vi "Property Name_Dots and Indents.vi"(11 "Property":string) -> (3 "Cluster":T1)   [LabVIEW 2023]
doc: "Bare property is when you have a subproperty (Bounds:Height) and you want just \"Height\"."
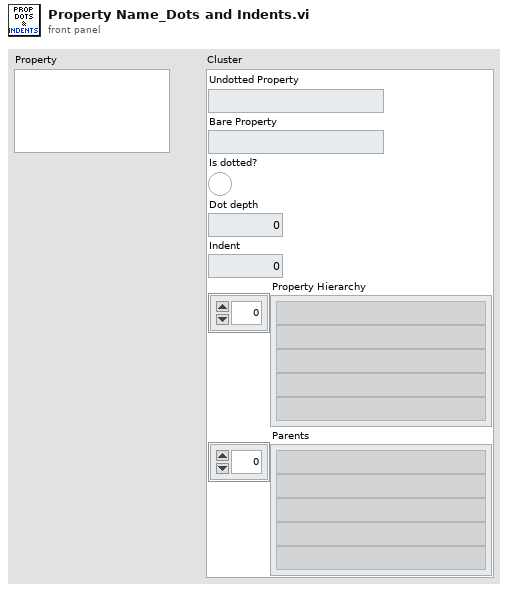
[diagram p1: front panel]
types:
  T1 = cluster{"Undotted Property":string, "Bare Property":string, "Is dotted?":bool, "Dot depth":i32, "Indent":i32, "Property Hierarchy":string[], "Parents":string[]}
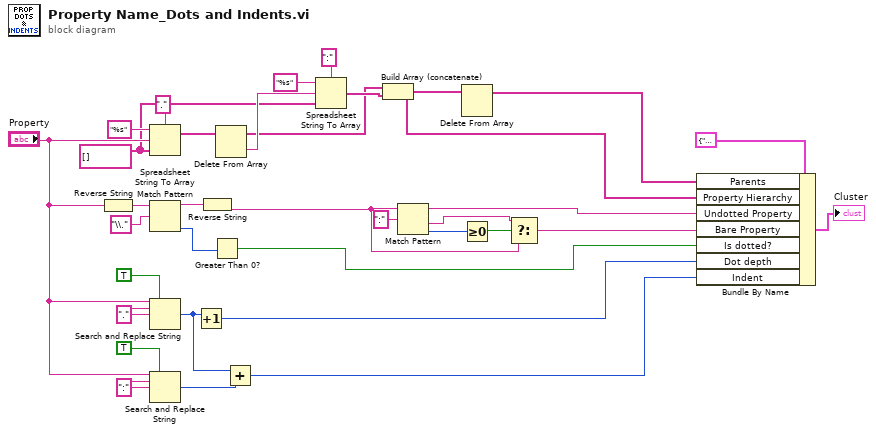
[diagram p0: block diagram]
diagram:
  w24 = ":" ("regular expression")
  w4 = string[] [] ("format string")
  w29 = "." ("regular expression")
  n1 = Reverse String(1:"Property") -> (0:w33:string)
  n2 = Spreadsheet String To Array(delimiter (Tab)=".", format string="%s", spreadsheet string="Property", array type (2D Dbl)=w4) -> (array=w8:string[])
  n3 = Match Pattern(string=w33, regular expression="\\.") -> (before substring=w31:string, offset past match=w30:i32)  [unwired: 1 in, 2 out]
  n4 = Search and Replace String(replace all?=TRUE ("replace all? (F)"), input string="Property", search string=w29, replace string=w29) -> (number of replacements=w23:i32)  [unwired: 4 in, 3 out]
  n5 = Search and Replace String(replace all?=TRUE ("replace all? (F)"), input string="Property", search string=w24, replace string=w24) -> (number of replacements=w22:i32)  [unwired: 4 in, 3 out]
  n6 = Increment(x=w23) -> (x+1=w11:i32)
  n7 = Reverse String(1:w31) -> (0:w13:string)
  n8 = Greater Than 0?(x=w30) -> (x > 0?=w12:bool)
  n9 = Delete From Array(array=w8) -> (deleted portion=w7:string, array with subset deleted=w3:string[])  [unwired: 2 in]
  n10 = Add(x=w23, y=w22) -> (x+y=w10:i32)
  n11 = Spreadsheet String To Array(delimiter (Tab)=":", format string="%s", spreadsheet string=w7, array type (2D Dbl)=w4) -> (array=w5:string[])
  n12 = Build Array (concatenate)(w3, w5) -> (w2:string[])
  n13 = Match Pattern(string=w13, regular expression=":") -> (after substring=w19:string, offset past match=w20:i32)  [unwired: 1 in, 2 out]
  n14 = Delete From Array(array=w2) -> (array with subset deleted=w1:string[])  [unwired: 2 in, 1 out]
  n15 = Greater Or Equal To 0?(x=w20) -> (x >= 0?=w18:bool)
  n16 = Select(t=w19, s=w18, f=w13) -> (s? t:f=w14:string)
  n17 = Bundle By Name(cluster=T1 {"Undotted Property"="c:d\n\n", "Bare Property"="d\n\n", "Is dotted?"=FALSE, "Dot depth"=1, "Indent"=1, "Property Hierarchy"=["c:d\n"], "Parents"=[]} ("Cluster"), "Parents"=w1, "Property Hierarchy"=w2, "Undotted Property"=w13, "Bare Property"=w14, "Is dotted?"=w12, "Dot depth"=w11, "Indent"=w10) -> (→"Cluster":T1)
